vi "BRig_dataCurrent_nReward_total.vi"() -> (2 "output_nReward_total":i32)   [LabVIEW 2014]
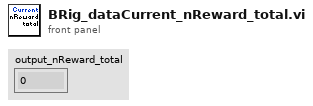
[diagram p1: front panel]
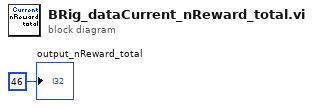
[diagram p0: block diagram]
diagram:
  "output_nReward_total" <- 46 ("output_iBlock")
